vi "Init.vi"(8 "error in (no error)":errorcluster, 11 "EEH - User Event in":refnum<class "EngineEventHandler-UserEvent.lvclass">) -> (0 "error out":errorcluster, 3 "EEH - User Event out":refnum<class "EngineEventHandler-UserEvent.lvclass">)   [LabVIEW 2020, in "GLF.lvlib" / "EngineEventHandler-UserEvent.lvclass"]
uses:
  EngineEventHandler-UserEvent.lvclass
  EngineEventHandler-UserEvent.lvclass/EngineEventHandler-UserEvent.ctl
  EngineEventInterface/EngineStopped-EventData--cluster.ctl
  EngineEventInterface/EngineEventInterface.lvclass
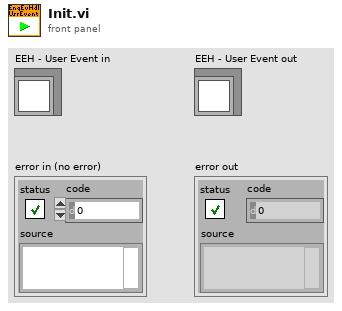
[diagram p1: front panel]
types:
  T1 = typedef "GLF.lvlib/EngineEventInterface.lvclass/EngineStopped-EventData--cluster.ctl" = cluster{"Error":errorcluster}
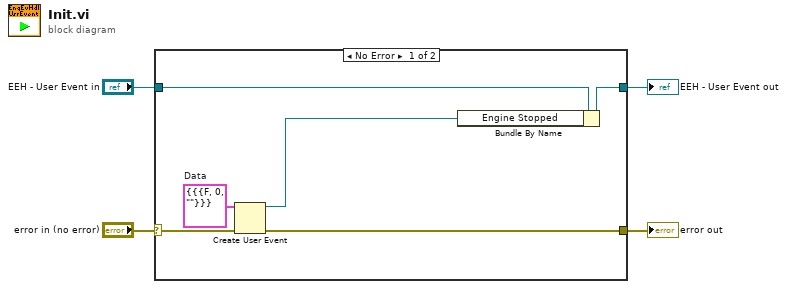
[diagram p0: block diagram]
diagram:
  n1 = case shown="No Error" "error in (no error)" {
    selector: "error in (no error)" -> [w9 w12]
    tunnel: [w7 w12] -> w3
    tunnel: [w8 w11] -> w1
    tunnel: "EEH - User Event in" -> [w10 w11]
    frame No Error {
      w6 = cluster{"Event Data":T1} {"Event Data"={"Error"={"status"=FALSE, "code"=0, "source"=""}}}  # Data
      n2 = Create User Event(user event datatype=w6, error in=w9) -> (user event=w5:refnum<user-event>, error out=w7:errorcluster)
      n3 = Bundle By Name(cluster=w10, "Engine Stopped"=w5) -> (w8:refnum<class "EngineEventHandler-UserEvent.lvclass">)
    }
    frame Error {
    }
  }
  "error out" <- w3
  "EEH - User Event out" <- w1
